vi "8HP_EnFlo_Specific.vi"(2 "Datalog file path (full)":path, 3 "COM port":refnum<visa-resource-name>, 4 "Log data stream":bool, 5 "Set data rate (Hz)":u8(ring)=14 items=["1", "2", "4", "5", "8", "10", "16", "20", "25", "32", "40", "50", "64", "80", "100", "125", "160", "200", "250", "320", "400", "500", "625", "800", "1000"], 6 "N samples":u32=1000, 7 "Command":T2="s") -> (0 "Error":errorcluster, 1 "All samples out":sgl[][](array[numeric]))   [LabVIEW 2020]
uses:
  ctls/8HP_Cmd (USB).ctl
  Globals/Meas_global.vi
panel:
  in  "Main":T1(tab)
  out "Serial number":sgl
  out "Subsystems ok":bool[](array[boolean])
  out "Pressure sensor values in range":bool[](array[boolean])
  out "Pressure sensor temperatures in range":bool[](array[boolean])
  out "Pressure sensor EEPROM checksums ok":bool[](array[boolean])
  out "P_raw_Azero":sgl[](array[numeric])
  out "n":u16
  out "Auto zero progBar":u16(slide) caption="Collecting samples, please maintain dP = 0" scale=0.0..1000.0
  in  "EEPROM array 2":u16[](array[numeric])
  in  "EEPROM array":sgl[](array[numeric])
  out "Chk ok":bool
  out "EEPROM Checksum":u8 format="%02x"
  out "received":bool
  out "Returned data rate (Hz)":u16
  out "sent":bool
  in  "Stop Data":bool
  out "Relative humidity (%)":sgl
  out "Env. sensor die temperature (deg C)":sgl
  out "External thermistor 0 temperature (deg C)":sgl
  out "Atmospheric pressure (mbar)":sgl
  out "Checksum ok":bool
  out "Gyration vector (deg / s)":sgl[](array[numeric])
  out "Acceleration vector (g)":sgl[](array[numeric])
  out "Pressures":sgl[][](graph)
  out "Stream enabled":bool
  out "External thermistor 1 temperature (deg C)":sgl
  # "Paul Nathan 10/2018"
  # "Output array order:\nP0 (Pa)\n  |\nP7 (Pa)\nT0 (deg C)\nT1 (deg C)\nP_atmos (mbar)\nT_env (deg C)\nRH (%)\nax (g)\nay (g)\naz (g)\nwx (deg / s)\nwy (deg / s)\nwz (deg / s)"
  # "Environmental sensor present"
  # "Inertial sensor present"
  # "Accelerometer self test pass"
  # "Gyroscope self test pass"
  # "External thermistor 0 value in range"
  # "External thermistor 1 value in range"
  # "MCU EEPROM checksum ok"
  # "Pressure sensor 0 value in range"
  # "Pressure sensor 1 value in range"
  # "Pressure sensor 2 value in range"
  # "Pressure sensor 3 value in range"
  # "Pressure sensor 4 value in range"
  # "Pressure sensor 5 value in range"
  # "Pressure sensor 6 value in range"
  # "Pressure sensor 7 value in range"
  # "Pressure sensor 0 temperature in range"
  # "Pressure sensor 1 temperature in range"
  # "Pressure sensor 2 temperature in range"
  # "Pressure sensor 3 temperature in range"
  # "Pressure sensor 4 temperature in range"
  # "Pressure sensor 5 temperature in range"
  # "Pressure sensor 6 temperature in range"
  # "Pressure sensor 7 temperature in range"
  # "Pressure sensor 0 EEPROM checksum okay"
  # "Pressure sensor 1 EEPROM checksum okay"
  # "Pressure sensor 2 EEPROM checksum okay"
  # "Pressure sensor 3 EEPROM checksum okay"
  # "Pressure sensor 4 EEPROM checksum okay"
  # "Pressure sensor 5 EEPROM checksum okay"
  # "Pressure sensor 6 EEPROM checksum okay"
  # "Pressure sensor 7 EEPROM checksum okay"
  # "of 1000"
  # "P0 raw auto-zero"
  # "P1 raw auto-zero"
  # "P2 raw auto-zero"
  # "P3 raw auto-zero"
  # "P4 raw auto-zero"
  # "P5 raw auto-zero"
  # "P6 raw auto-zero"
  # "P7 raw auto-zero"
  # "Power-up defaults"
  # "Data rate (Hz)"
  # "TTL streaming"
  # "USB streaming"
  # "TTL stream contains full data"
  # "Accelerometer range mode"
  # "Gyroscope range mode"
  # "IMU rate mode"
  # "P0 raw auto-zero"
  # "P1 raw auto-zero"
  # "P2 raw auto-zero"
  # "P3 raw auto-zero"
  # "P4 raw auto-zero"
  # "P5 raw auto-zero"
  # "P6 raw auto-zero"
  # "P7 raw auto-zero"
  # "Atmospheric pressure offset (Pa)"
  # "External thermistor 0 temperature offset (deg C)"
  # "External thermistor 1 temperature offset (deg C)"
  # "Serial number"
  # "Baud rate (bps)"
  # "Accelerometer vector magnitude scale factor"
  # "Gyroscope x component offset (deg / s)"
  # "Gyroscope y component offset (deg / s)"
  # "Gyroscope z component offset (deg / s)"
  # "w_x"
  # "w_y"
  # "w_z"
  # "a_x"
  # "a_y"
  # "a_z"
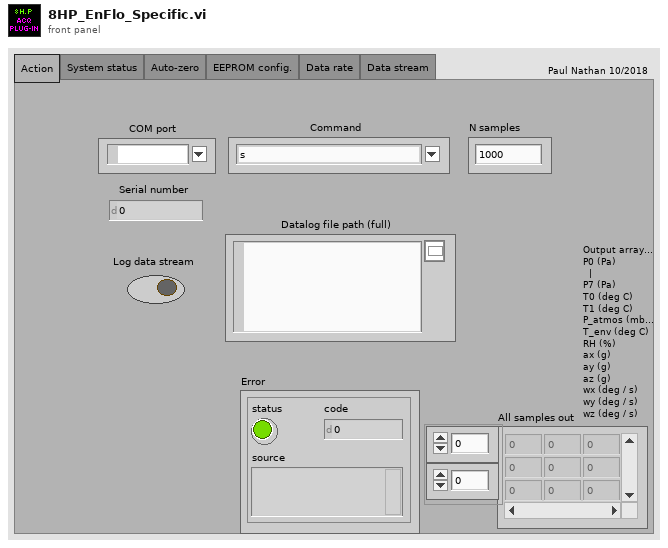
[diagram p1: front panel]
types:
  T1 = enum32{"Action", "System status", "Auto-zero", "EEPROM config.", "Data rate", "Data stream"}
  T2 = typedef "8HP_Cmd (USB).ctl" = string
  T3 = enum16{"open", "replace", "create", "open or create", "replace or create", "replace or create with confirmation"}
  T4 = typedef "Rendezvous RefNum" = refnum<k1>
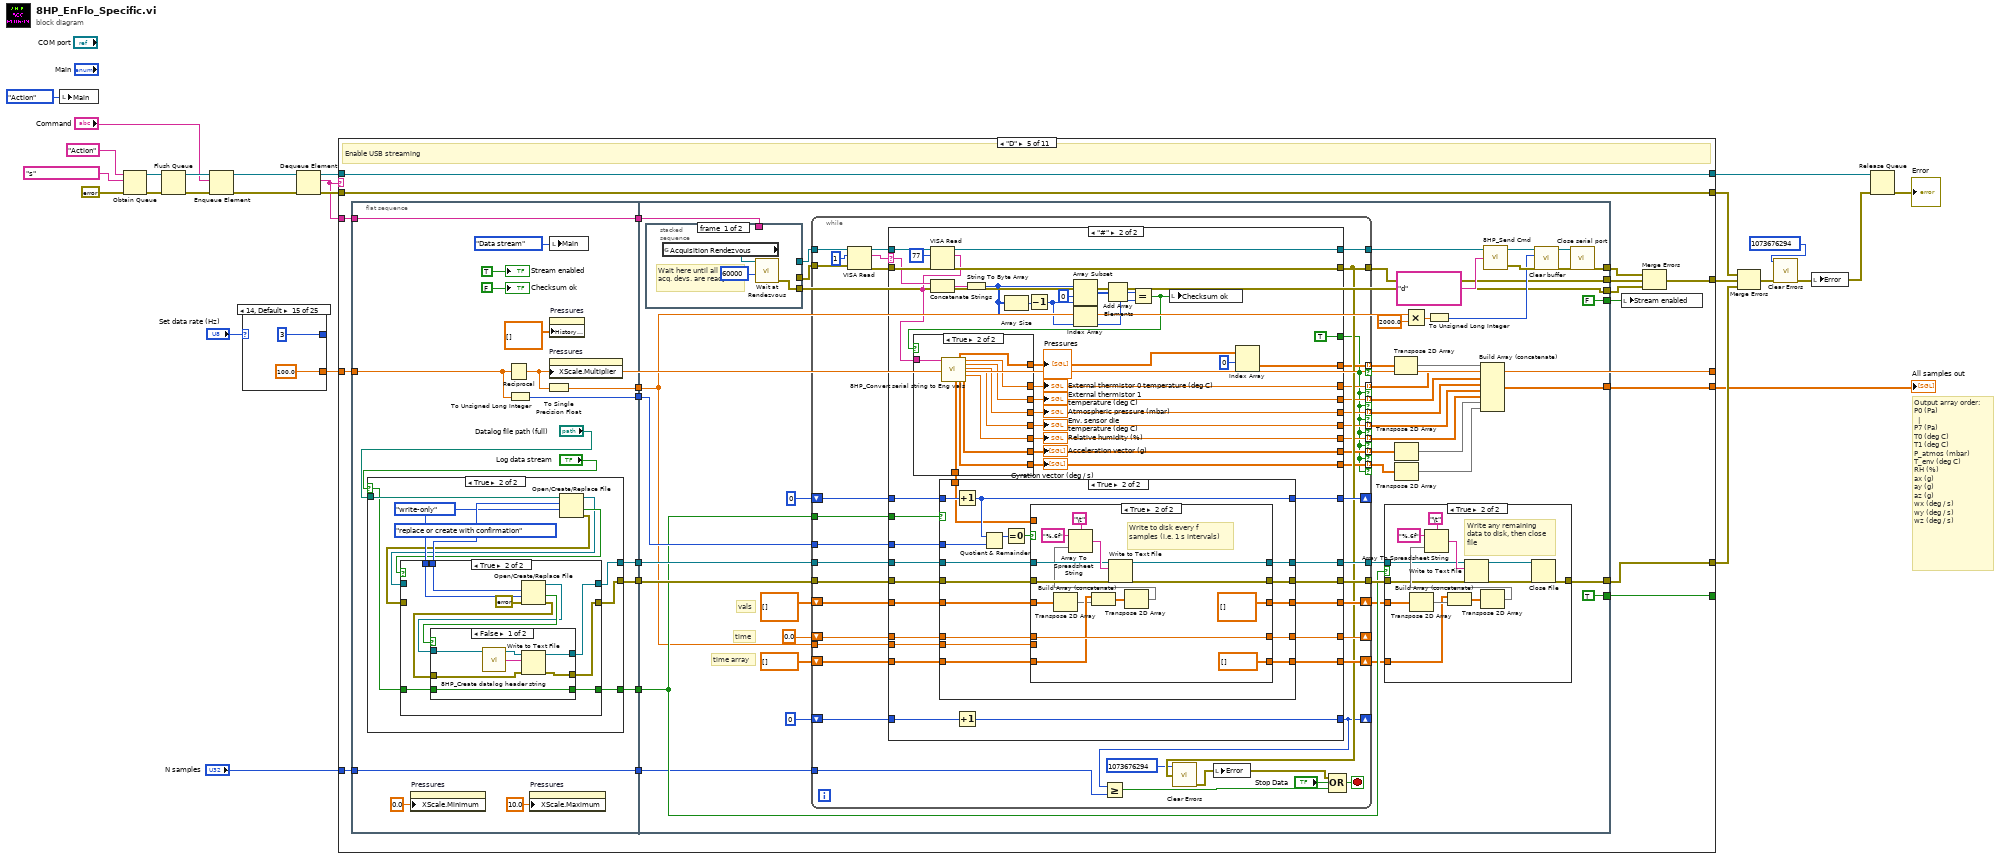
[diagram p0: block diagram]
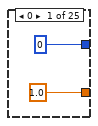
[diagram p2: hidden frame]
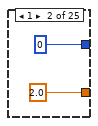
[diagram p3: hidden frame]
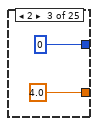
[diagram p4: hidden frame]
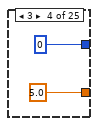
[diagram p5: hidden frame]
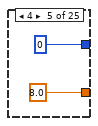
[diagram p6: hidden frame]
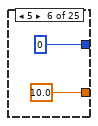
[diagram p7: hidden frame]
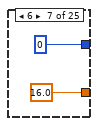
[diagram p8: hidden frame]
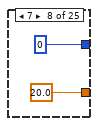
[diagram p9: hidden frame]
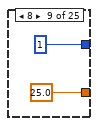
[diagram p10: hidden frame]
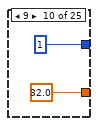
[diagram p11: hidden frame]
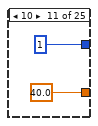
[diagram p12: hidden frame]
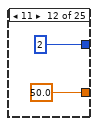
[diagram p13: hidden frame]
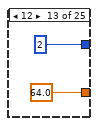
[diagram p14: hidden frame]
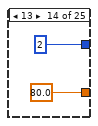
[diagram p15: hidden frame]
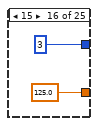
[diagram p16: hidden frame]
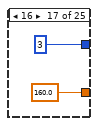
[diagram p17: hidden frame]
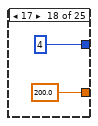
[diagram p18: hidden frame]
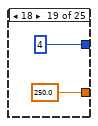
[diagram p19: hidden frame]
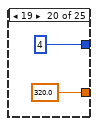
[diagram p20: hidden frame]
diagram:
  # "Output array order:\nP0 (Pa)\n  |\nP7 (Pa)\nT0 (deg C)\nT1 (deg C)\nP_atmos (mbar)\nT_env (deg C)\nRH (%)\nax (g)\nay (g)\naz (g)\nwx (deg / s)\nwy (deg / s)\nwz (deg / s)"
  n1 = local write "Main"(T1."Action" ("Main")) -> ()
  n2 = Obtain Queue(name (unnamed)="Action", element data type=T2 "s" ("Combo Box"), error in (no error)=errorcluster {"status"=FALSE, "code"=0, "source"=""}) -> (queue out=w24:refnum<queue>, error out=w25:errorcluster)  [unwired: 2 in, 1 out]
  n3 = Flush Queue(queue=w24, error in (no error)=w25) -> (queue out=w17:refnum<queue>, error out=w16:errorcluster)  [unwired: 1 out]
  n4 = Enqueue Element(queue=w17, element="Command", error in (no error)=w16) -> (queue out=w19:refnum<queue>, error out=w18:errorcluster)  [unwired: 1 in, 1 out]
  n5 = case shown="14, Default" "Set data rate (Hz)" {
    tunnel: [1.0 2.0 4.0 5.0 8.0 10.0 16.0 20.0 25.0 32.0 40.0 50.0 64.0 80.0 100.0 125.0 160.0 200.0 250.0 320.0 400.0 500.0 625.0 800.0 1000.0] -> w4
    tunnel: [u8 0 u8 0 u8 0 u8 0 u8 0 u8 0 u8 0 u8 0 u8 1 u8 1 u8 1 u8 2 u8 2 u8 2 u8 3 u8 3 u8 3 u8 4 u8 4 u8 4 u8 5 u8 5 u8 6 u8 6 u8 6] -> _
    frame 0 {
    }
    frame 1 {
    }
    frame 2 {
    }
    frame 3 {
    }
    frame 4 {
    }
    frame 5 {
    }
    frame 6 {
    }
    frame 7 {
    }
    frame 8 {
    }
    frame 9 {
    }
    frame 10 {
    }
    frame 11 {
    }
    frame 12 {
    }
    frame 13 {
    }
    frame 14, Default {
    }
    frame 15 {
    }
    frame 16 {
    }
    frame 17 {
    }
    frame 18 {
    }
    frame 19 {
    }
    frame 20 {
    }
    frame 21 {
    }
    frame 22 {
    }
    frame 23 {
    }
    frame 24 {
    }
  }
  n6 = Dequeue Element(queue=w19, error in (no error)=w18) -> (queue out=w14:refnum<queue>, element=w12:T2, error out=w13:errorcluster)  [unwired: 1 in, 1 out]
  n7 = case shown="\"D\"" w12 {
    tunnel: [w83 w124 w163 w239 w317 w607 w633 w716 w756 FALSE FALSE] -> _
    tunnel: w14 -> [w82 w123 w162 w238 w316 w609 w635 w718 w755 w780 w785]
    tunnel: [w82 w123 w162 w238 w316 w609 w635 w718 w755 w780 w785] -> w6
    tunnel: w13 -> [w81 w122 w161 w237 w315 w608 w636 w719 w754 w779 w784]
    tunnel: [w81 w122 w161 w237 w315 w608 w636 w719 w754 w779 w784] -> w11
    tunnel: w12 -> [w80 w121 w160 w236 w314 w611 w641 w724 w753 _ _]
    tunnel: [w78 w119 w158 w233 w300 w610 w634 w717 w751 errorcluster {"status"=FALSE, "code"=0, "source"=""} ("Error out") errorcluster {"status"=FALSE, "code"=0, "source"=""} ("Error out")] -> w10
    tunnel: [_ _ _ _ w312 _ _ _ _ _ _] -> w9
    tunnel: w4 -> [w77 w118 w157 w232 w305 w605 _ _ w750 w776 w781]
    tunnel: [w77 w118 w157 w232 w305 w605 w637 w720 w750 w776 w781] -> _
    tunnel: [_ _ _ _ w304 _ _ _ _ _ _] -> w2
    tunnel: "N samples" -> [_ _ _ _ w298 _ _ _ _ _ _]
    frame "S", "s" {
      # "Perform self-test and retrieve status bytes, Retrieve status bytes"
      n8 = flat-sequence {
        tunnel: w80 -> [w86]
        tunnel: [w86] -> w79
        tunnel: [TRUE] -> w83
        tunnel: w79 -> [w92]
        tunnel: [w87] -> w78
        frame #0 {
          w85 = bool[] [] ("Pressure sensor EEPROM checksums ok")
          n9 = local write "Main"(T1."System status" ("Main")) -> ()
          "Pressure sensor EEPROM checksums ok" <- w85
          "Pressure sensor temperatures in range" <- w85
          "Pressure sensor values in range" <- w85
          "Subsystems ok" <- w85
        }
        frame #1 {
          w97 = 1 ("length (rest)")
          w105 = u8 0 ("byte count")
          n10 = local read "COM port"() -> (w93:refnum<visa-resource-name>)
          n11 = call "Open serial port.vi"("timeout (ms)"=u32 5000, "VISA resource name"=w93) -> ("Error out"=w115:errorcluster, "VISA resource name out"=w116:refnum<visa-resource-name>)  [unwired: 8 in]
          n12 = call "8HP_Send Cmd.vi"("Error In"=w115, "Operation"=w92, "Port"=w116) -> ("Error Out"=w113:errorcluster, "Port out"=w114:refnum<visa-resource-name>)  [unwired: 1 in]
          n13 = VISA Read(VISA resource name=w114, byte count=u32 4, error in (no error)=w113) -> (VISA resource name out=w111:refnum<visa-resource-name>, read buffer=w100:string, error out=w110:errorcluster)  [unwired: 1 out]
          n14 = call "Close serial port.vi"("Error in"=w110, "VISA resource name"=w111) -> ("Error out"=w87:errorcluster)  [unwired: 9 in]
          n15 = String Subset(string=w100, offset (0)=0, length (rest)=w97) -> (substring=w109:string)
          n16 = String Subset(string=w100, offset (0)=1, length (rest)=w97) -> (substring=w108:string)
          n17 = String Subset(string=w100, offset (0)=2 ("length (rest)"), length (rest)=w97) -> (substring=w107:string)
          n18 = String Subset(string=w100, offset (0)=3, length (rest)=w97) -> (substring=w106:string)
          n19 = Type Cast(type=w105, x=w109) -> (*(type *) &x=w104:u8)
          n20 = Type Cast(type=w105, x=w108) -> (*(type *) &x=w103:u8)
          n21 = Type Cast(type=w105, x=w107) -> (*(type *) &x=w102:u8)
          n22 = Type Cast(type=w105, x=w106) -> (*(type *) &x=w101:u8)
          n23 = Number To Boolean Array(number=w104) -> (Boolean array=w91:bool[])
          n24 = Number To Boolean Array(number=w103) -> (Boolean array=w90:bool[])
          n25 = Number To Boolean Array(number=w102) -> (Boolean array=w89:bool[])
          n26 = Number To Boolean Array(number=w101) -> (Boolean array=w88:bool[])
          n27 = local write "Pressure sensor EEPROM checksums ok"(w91) -> ()
          n28 = local write "Pressure sensor temperatures in range"(w90) -> ()
          n29 = local write "Pressure sensor values in range"(w89) -> ()
          n30 = local write "Subsystems ok"(w88) -> ()
        }
      }
    }
    frame "Z", "z" {
      # "Perform permanent auto-zero (write values to EEPROM), Perform temporary auto-zero"
      n31 = flat-sequence {
        tunnel: w121 -> [w128]
        tunnel: [w128] -> w120
        tunnel: [TRUE] -> w124
        tunnel: w120 -> [w135]
        tunnel: [w131] -> w119
        frame #0 {
          n32 = local write "Main"(T1."Auto-zero" ("Main")) -> ()
          "P_raw_Azero" <- sgl[] [] ("P_raw_Azero")
          "Auto zero progBar" <- u16 0 ("Collecting samples, please maintain dP = 0")
        }
        frame #1 {
          n33 = local read "COM port"() -> (w136:refnum<visa-resource-name>)
          n34 = call "Open serial port.vi"("timeout (ms)"=u32 16000, "VISA resource name"=w136) -> ("Error out"=w143:errorcluster, "VISA resource name out"=w144:refnum<visa-resource-name>)  [unwired: 8 in]
          n35 = call "8HP_Send Cmd.vi"("Error In"=w143, "Operation"=w135, "Port"=w144) -> ("Error Out"=w141:errorcluster, "Port out"=w142:refnum<visa-resource-name>)  [unwired: 1 in]
          n36 = VISA Read(VISA resource name=w142, byte count=u32 32, error in (no error)=w141) -> (VISA resource name out=w139:refnum<visa-resource-name>, read buffer=w132:string, error out=w138:errorcluster)  [unwired: 1 out]
          n37 = for {
            N: 1000 -> [_]
            shift-right: [w146] -> _
            shift-left: u16 0 -> [w147]
            n38 = Increment(x=w147) -> (x+1=w146:u16)
            "n" <- w146
            n39 = Wait (ms)(milliseconds to wait=u32 10) -> ()  [unwired: 1 out]
            n40 = local write "Auto zero progBar"(w146) -> ()
          }
          n41 = for {
            N: 8 -> [_]
            tunnel: [w150] -> w134 mode=indexing
            tunnel: w132 -> [w149]
            i -> [w156]
            w154 = 4 ("x")
            # "to BE"
            n42 = Multiply(x=w154, y=w156) -> (x*y=w155:i32)
            n43 = String Subset(string=w149, offset (0)=w155, length (rest)=w154) -> (substring=w153:string)
            n44 = Reverse String(1:w153) -> (0:w152:string)
            n45 = Type Cast(type=sgl 0.0 ("byte count"), x=w152) -> (*(type *) &x=w150:sgl)
          }
          n46 = call "Close serial port.vi"("Error in"=w138, "VISA resource name"=w139) -> ("Error out"=w131:errorcluster)  [unwired: 9 in]
          n47 = local write "P_raw_Azero"(w134) -> ()
        }
      }
    }
    frame "R" {
      # "Read all EEPROM values"
      n48 = flat-sequence {
        tunnel: w160 -> [w167]
        tunnel: [w167] -> w159
        tunnel: [TRUE] -> w163
        tunnel: w159 -> [w202]
        tunnel: [w191] -> w158
        frame #0 {
          n49 = local write "EEPROM array"(sgl[] [] ("EEPROM array")) -> ()
          n50 = local write "EEPROM array 2"(u16[] [] ("EEPROM array 2")) -> ()
          n51 = local write "Main"(T1."EEPROM config." ("Main")) -> ()
        }
        frame #1 {
          # "to BE"
          n52 = local read "COM port"() -> (w203:refnum<visa-resource-name>)
          n53 = call "Open serial port.vi"("timeout (ms)"=u32 5000, "VISA resource name"=w203) -> ("Error out"=w210:errorcluster, "VISA resource name out"=w211:refnum<visa-resource-name>)  [unwired: 8 in]
          n54 = call "8HP_Send Cmd.vi"("Error In"=w210, "Operation"=w202, "Port"=w211) -> ("Error Out"=w208:errorcluster, "Port out"=w209:refnum<visa-resource-name>)  [unwired: 1 in]
          n55 = VISA Read(VISA resource name=w209, byte count=u32 78, error in (no error)=w208) -> (VISA resource name out=w206:refnum<visa-resource-name>, read buffer=w174:string, error out=w205:errorcluster)  [unwired: 1 out]
          n56 = String To Byte Array(string=w174) -> (unsigned byte array=w194:u8[])
          n57 = call "Close serial port.vi"("Error in"=w205, "VISA resource name"=w206) -> ("Error out"=w191:errorcluster)  [unwired: 9 in]
          n58 = String Subset(string=w174, offset (0)=0, length (rest)=56 ("length (rest)")) -> (substring=w189:string)
          n59 = String Subset(string=w174, offset (0)=64, length (rest)=12 ("length (rest)")) -> (substring=w184:string)
          n60 = String Subset(string=w174, offset (0)=56, length (rest)=2 ("length (rest)")) -> (substring=w173:string)
          n61 = String Subset(string=w174, offset (0)=58, length (rest)=6 ("length (rest)")) -> (substring=w168:string)
          n62 = Array Size(array=w194) -> (size(s)=w196:i32)
          n63 = Decrement(x=w196) -> (x-1=w195:i32)
          n64 = for {
            N: 14 -> [_]
            tunnel: [w224] -> w183 mode=indexing
            tunnel: w189 -> [w223]
            i -> [w228]
            w226 = 4 ("x")
            # "to BE"
            n65 = Multiply(x=w226, y=w228) -> (x*y=w227:i32)
            n66 = String Subset(string=w223, offset (0)=w227, length (rest)=w226) -> (substring=w222:string)
            n67 = Reverse String(1:w222) -> (0:w221:string)
            n68 = Type Cast(type=sgl 0.0 ("byte count"), x=w221) -> (*(type *) &x=w224:sgl)
          }
          n69 = for {
            N: 3 -> [_]
            tunnel: [w216] -> w182 mode=indexing
            tunnel: w184 -> [w215]
            i -> [w220]
            w218 = 4 ("x")
            # "to BE"
            n70 = Multiply(x=w218, y=w220) -> (x*y=w219:i32)
            n71 = String Subset(string=w215, offset (0)=w219, length (rest)=w218) -> (substring=w214:string)
            n72 = Reverse String(1:w214) -> (0:w213:string)
            n73 = Type Cast(type=sgl 0.0 ("byte count"), x=w213) -> (*(type *) &x=w216:sgl)
          }
          n74 = Index Array(array=w194, index=77) -> (element=w198:u8)
          n75 = Array Subset(array=w194, index=0, length=w195) -> (w192:u8[])
          n76 = Reverse String(1:w173) -> (0:w180:string)
          n77 = Add Array Elements(numeric array=w192) -> (sum=w193:u8)
          n78 = Type Cast(type=u16 0 ("byte count"), x=w180) -> (*(type *) &x=w172:u16)
          n79 = String To Byte Array(string=w168) -> (unsigned byte array=w171:u8[])
          n80 = To Unsigned Word Integer(number=w171) -> (unsigned 16bit integer=w169:u16[])
          n81 = Equal?(x=w198, y=w193) -> (x = y?=w200:bool)
          n82 = Build Array (concatenate)(w183, w182) -> (w181:sgl[])
          n83 = Build Array (concatenate)(w172, w169) -> (w170:u16[])
          n84 = local write "EEPROM array"(w181) -> ()
          n85 = local write "EEPROM array 2"(w170) -> ()
          n86 = local write "EEPROM Checksum"(w198) -> ()
          n87 = local write "Chk ok"(w200) -> ()
        }
      }
    }
    frame "W" {
      # "Write all EEPROM values (including new checksum)"
      n88 = flat-sequence {
        tunnel: w236 -> [w252]
        tunnel: [w252] -> w235
        tunnel: [w246] -> w234
        tunnel: [w245] -> w231
        tunnel: [w241] -> w230
        tunnel: [w242] -> w229
        tunnel: [TRUE] -> w239
        tunnel: w235 -> [w280]
        tunnel: w234 -> [w274]
        tunnel: [w272] -> w233
        tunnel: w231 -> [w261]
        tunnel: w230 -> [w258]
        tunnel: w229 -> [w256]
        frame #0 {
          n89 = local write "Main"(T1."EEPROM config." ("Main")) -> ()
          n90 = Split 1D Array(array="EEPROM array", index=14) -> (first subarray=w246:sgl[], second subarray=w245:sgl[])
          n91 = Split 1D Array(array="EEPROM array 2", index=1) -> (first subarray=w244:u16[], second subarray=w243:u16[])
          n92 = Index Array(array=w244, index=0) -> (element=w241:u16)
          n93 = To Unsigned Byte Integer(number=w243) -> (unsigned 8bit integer=w242:u8[])
        }
        frame #1 {
          # "to LE"
          n94 = local read "COM port"() -> (w281:refnum<visa-resource-name>)
          n95 = for {
            N: 14 -> [_]
            tunnel: w274 -> [w294] mode=indexing
            shift-right: [w295] -> w267
            shift-left: "" -> [w296]
            # "to LE"
            n96 = Type Cast(type="", x=w294) -> (*(type *) &x=w293:string)
            n97 = Reverse String(1:w293) -> (0:w292:string)
            n98 = Concatenate Strings(w296, w292) -> (w295:string)
          }
          n99 = for {
            N: 3 -> [_]
            tunnel: w261 -> [w288] mode=indexing
            shift-right: [w289] -> w254
            shift-left: "" -> [w290]
            # "to LE"
            n100 = Type Cast(type="", x=w288) -> (*(type *) &x=w287:string)
            n101 = Reverse String(1:w287) -> (0:w286:string)
            n102 = Concatenate Strings(w290, w286) -> (w289:string)
          }
          n103 = Type Cast(type="", x=w258) -> (*(type *) &x=w260:string)
          n104 = Reverse String(1:w260) -> (0:w257:string)
          n105 = Byte Array To String(unsigned byte array=w256) -> (string=w253:string)
          n106 = call "Open serial port.vi"("timeout (ms)"=u32 5000, "VISA resource name"=w281) -> ("Error out"=w283:errorcluster, "VISA resource name out"=w284:refnum<visa-resource-name>)  [unwired: 8 in]
          n107 = Type Cast(type="", x=u8 0) -> (*(type *) &x=w255:string)
          n108 = Concatenate Strings(w267, w257, w253, w254, w255) -> (w264:string)
          n109 = String To Byte Array(string=w264) -> (unsigned byte array=w268:u8[])
          n110 = Add Array Elements(numeric array=w268) -> (sum=w273:u8)
          "EEPROM Checksum" <- w273
          n111 = Type Cast(type="", x=w273) -> (*(type *) &x=w276:string)
          n112 = Concatenate Strings(w264, w276) -> (w271:string)
          n113 = call "8HP_Send Cmd + Data.vi"("Error In"=w283, "Data"=w271, "Operation"=w280, "Port"=w284) -> ("Error Out"=w269:errorcluster, "Port out"=w270:refnum<visa-resource-name>)  [unwired: 1 in]
          n114 = call "Close serial port.vi"("Error in"=w269, "VISA resource name"=w270) -> ("Error out"=w272:errorcluster)  [unwired: 9 in]
          "Chk ok" <- TRUE ("Chk ok")
        }
      }
    }
    frame "D" {
      # "Enable USB streaming"
      n115 = flat-sequence {
        tunnel: w314 -> [w334]
        tunnel: [w334] -> w313
        tunnel: [w331] -> w311
        tunnel: [w330] -> w310
        tunnel: [w329] -> w309
        tunnel: w305 -> [w320]
        tunnel: [w327] -> w308
        tunnel: [w323] -> w307
        tunnel: [w321] -> w299
        tunnel: w298 -> [w321]
        tunnel: [TRUE] -> w317
        tunnel: w313 -> [w389]
        tunnel: [w416] -> w302
        tunnel: [w415] -> w312
        tunnel: w311 -> [w412]
        tunnel: w310 -> [w411]
        tunnel: w309 -> [w413]
        tunnel: w308 -> [w395]
        tunnel: w307 -> [w405]
        tunnel: [FALSE] -> w306
        tunnel: [w385] -> w304
        tunnel: [w373] -> w301
        tunnel: [w376] -> w303
        tunnel: w299 -> [w375]
        frame #0 {
          n116 = case shown="True" "Log data stream" {
            selector: "Log data stream" -> [w335 w338]
            tunnel: "Datalog file path (full)" -> [_ w347]
            tunnel: [refnum<file> refnum ("refnum out") w344] -> w331
            tunnel: [errorcluster {"status"=FALSE, "code"=0, "source"=""} ("error out") w343] -> w330
            tunnel: [w335 w339] -> w323
            frame False {
            }
            frame True {
              w345 = enum16{"read/write", "read-only", "write-only"}."write-only" ("access (0:read/write)")
              w346 = T3."replace or create with confirmation" ("operation (0:open)")
              n117 = Open/Create/Replace File(file path (use dialog)=w347, operation (0:open)=w346, access (0:read/write)=w345) -> (refnum out=w340:refnum<file>, cancelled=w342:bool, error out=w341:errorcluster)  [unwired: 3 in]
              n118 = case shown="True" w342 {
                tunnel: w346 -> [_ w363]
                tunnel: w345 -> [_ w362]
                tunnel: w341 -> [w351 _]
                tunnel: [w349 w357] -> w344
                tunnel: [w350 w358] -> w343
                tunnel: w340 -> [w352 _]
                tunnel: [w348 w355] -> w339
                tunnel: w338 -> [w348 w354]
                frame False {
                  n119 = call "8HP_Create datalog header string.vi"() -> ("Datalog header string"=w353:string)  [unwired: 1 in]
                  n120 = Write to Text File(file (use dialog)=w352, text=w353, error in=w351) -> (refnum out=w349:refnum<file>, error out=w350:errorcluster)  [unwired: 1 in, 1 out]
                }
                frame True {
                  n121 = Open/Create/Replace File(error in=errorcluster {"status"=FALSE, "code"=0, "source"=""}, operation (0:open)=w363, access (0:read/write)=w362) -> (refnum out=w360:refnum<file>, cancelled=w361:bool, error out=w359:errorcluster)  [unwired: 3 in]
                  n122 = case shown="False" w361 {
                    tunnel: w360 -> [w368 _]
                    tunnel: w359 -> [w367 _]
                    tunnel: [w366 errorcluster {"status"=FALSE, "code"=0, "source"=""} ("error out")] -> w358
                    tunnel: [w365 refnum<file> refnum ("t")] -> w357
                    tunnel: [w364 w370] -> w355
                    tunnel: w354 -> [w364 _]
                    frame False {
                      n123 = call "8HP_Create datalog header string.vi"() -> ("Datalog header string"=w369:string)  [unwired: 1 in]
                      n124 = Write to Text File(file (use dialog)=w368, text=w369, error in=w367) -> (refnum out=w365:refnum<file>, error out=w366:errorcluster)  [unwired: 1 in, 1 out]
                    }
                    frame True {
                      w370 = FALSE ("Log data stream")
                      n125 = local write "Log data stream"(w370) -> ()
                    }
                  }
                }
              }
            }
          }
          n126 = property on="Pressures" class="WFChart (strict)"("XScale.Minimum"=0.0 ("X Scale.Range:Minimum")) -> ()  [unwired: 2 in, 2 out]
          n127 = Reciprocal(x=w320) -> (1/x=w328:dbl)
          n128 = To Unsigned Long Integer(number=w320) -> (unsigned 32bit integer=w329:u32)
          n129 = property on="Pressures" class="WFChart (strict)"("XScale.Maximum"=10.0 ("X Scale.Range:Minimum")) -> ()  [unwired: 2 in, 2 out]
          n130 = To Single Precision Float(number=w328) -> (single precision float=w327:sgl)
          n131 = property on="Pressures" class="WFChart (strict)"("XScale.Multiplier"=w328) -> ()  [unwired: 2 in, 2 out]
          n132 = local write "Main"(T1."Data stream" ("Main")) -> ()
          n133 = property on="Pressures" class="WFChart (strict)"("History Data"=sgl[][] []) -> ()  [unwired: 2 in, 2 out]
          "Checksum ok" <- FALSE ("Checksum ok")
          "Stream enabled" <- TRUE ("Stream enabled")
        }
        frame #1 {
          # "vals"
          # "time"
          # "time array"
          n134 = stacked-sequence {
            tunnel: [_ w425] -> w404
            tunnel: [_ w423] -> w403
            tunnel: w389 -> [_ w421]
            tunnel: [w419 _] -> w373
            frame #0 {
              # "Wait here until all acq. devs. are ready."
              n135 = global read "Meas_global.vi" "Acquisition Rendezvous"() -> (w420:T4)
              n136 = call <vilib>:"Wait at Rendezvous.vi"("ms timeout (-1)"=60000, "rendezvous"=w420) -> ("error out"=w419:errorcluster)  [unwired: 3 in, 2 out]
            }
            frame #1 {
              n137 = local read "COM port"() -> (w427:refnum<visa-resource-name>)
              n138 = call "Open serial port.vi"("timeout (ms)"=u32 5000, "VISA resource name"=w427) -> ("Error out"=w424:errorcluster, "VISA resource name out"=w426:refnum<visa-resource-name>)  [unwired: 8 in]
              n139 = call "8HP_Send Cmd.vi"("Error In"=w424, "Operation"=w421, "Port"=w426) -> ("Error Out"=w423:errorcluster, "Port out"=w425:refnum<visa-resource-name>)  [unwired: 1 in]
            }
          }
          n140 = while {
            tunnel: [w457] -> w376
            tunnel: w404 -> [w459]
            tunnel: [w477] -> w402
            shift-right: [w473] -> _
            shift-left: u32 0 -> [w474]
            tunnel: w413 -> [w472]
            tunnel: w412 -> [w471]
            tunnel: w411 -> [w470]
            tunnel: [w469] -> w410
            tunnel: [w468] -> w409
            shift-right: [w467] -> w392
            shift-left: sgl[][] [] -> [w466]
            shift-right: [w463] -> _
            shift-left: sgl 0.0 ("Numeric") -> [w465]
            tunnel: w395 -> [w464]
            shift-right: [w461] -> w391
            shift-left: sgl[] [] -> [w462]
            tunnel: w405 -> [w460]
            tunnel: w403 -> [w458]
            tunnel: [w454] -> w384 mode=indexing if=w446
            tunnel: [w453] -> w383 mode=indexing if=w446
            tunnel: [w452] -> w382 mode=indexing if=w446
            tunnel: [w451] -> w381 mode=indexing if=w446
            tunnel: [w450] -> w380 mode=indexing if=w446
            tunnel: [w449] -> w377 mode=indexing if=w446
            tunnel: [w448] -> w378 mode=indexing if=w446
            tunnel: [w447] -> w379 mode=indexing if=w446
            tunnel: w375 -> [w444]
            shift-right: [w442] -> _
            shift-left: u32 0 -> [w445]
            stop <- w475 stop-if-true
            n141 = VISA Read(VISA resource name=w459, byte count=u32 1, error in (no error)=w458) -> (VISA resource name out=w479:refnum<visa-resource-name>, read buffer=w480:string, error out=w478:errorcluster)  [unwired: 1 out]
            n142 = case shown="\"#\"" w480 {
              selector: w480 -> [_ w531]
              tunnel: w479 -> [w490 w535]
              tunnel: [w491 w533] -> w457
              tunnel: w478 -> [w491 w536]
              tunnel: [w490 w534] -> w477
              tunnel: w474 -> [w489 w521]
              tunnel: [w489 w520] -> w473
              tunnel: w472 -> [_ w519]
              tunnel: w471 -> [w488 w518]
              tunnel: w470 -> [w487 w517]
              tunnel: [w487 w516] -> w469
              tunnel: [w488 w515] -> w468
              tunnel: [w486 w514] -> w467
              tunnel: w466 -> [w486 w513]
              tunnel: w465 -> [w485 w512]
              tunnel: w464 -> [_ w511]
              tunnel: [w485 w510] -> w463
              tunnel: w462 -> [w484 w509]
              tunnel: [w484 w508] -> w461
              tunnel: w460 -> [_ w507]
              tunnel: [_ w506] -> w454
              tunnel: [FALSE TRUE] -> w446
              tunnel: [_ w492] -> w453
              tunnel: [_ w493] -> w452
              tunnel: [_ w494] -> w451
              tunnel: [_ w500] -> w450
              tunnel: [_ w499] -> w449
              tunnel: [_ w498] -> w448
              tunnel: [_ w497] -> w447
              tunnel: w445 -> [w482 w496]
              tunnel: [w482 w495] -> w442
              frame Default {
              }
              frame "#" {
                n143 = VISA Read(VISA resource name=w535, byte count=u32 77, error in (no error)=w536) -> (VISA resource name out=w534:refnum<visa-resource-name>, read buffer=w522:string, error out=w533:errorcluster)  [unwired: 1 out]
                n144 = Concatenate Strings(w531, w522) -> (w523:string)
                n145 = Increment(x=w496) -> (x+1=w495:u32)
                n146 = String To Byte Array(string=w523) -> (unsigned byte array=w526:u8[])
                n147 = Array Size(array=w526) -> (size(s)=w529:i32)
                n148 = Decrement(x=w529) -> (x-1=w525:i32)
                n149 = Array Subset(array=w526, index=0, length=w525) -> (w530:u8[])
                n150 = Index Array(array=w526, index=w525) -> (element=w524:u8)
                n151 = Add Array Elements(numeric array=w530) -> (sum=w527:u8)
                n152 = Equal?(x=w527, y=w524) -> (x = y?=w502:bool)
                n153 = case shown="True" w502 {
                  tunnel: w522 -> [_ w556]
                  tunnel: [w546 w555] -> w492
                  tunnel: [w546 w554] -> w493
                  tunnel: [w546 w553] -> w500
                  tunnel: [w546 w552] -> w499
                  tunnel: [w544 w551] -> w498
                  tunnel: [w544 w550] -> w497
                  tunnel: [w541 w549] -> w505
                  tunnel: [w546 w548] -> w494
                  tunnel: [w537 w547] -> w503
                  frame False {
                    (unwired) 3 ("dimension size")
                    w546 = sgl nan ("Atmospheric pressure (mbar)")
                    n154 = Initialize Array(sgl nan ("element"), 8 ("dimension size")) -> (w540:sgl[])
                    n155 = Initialize Array(sgl nan ("element")) -> (w544:sgl[])  [unwired: 1 in]
                    n156 = Initialize Array(sgl nan ("element"), 19 ("dimension size")) -> (w541:sgl[])
                    n157 = Build Array(w540) -> (w537:sgl[][])
                  }
                  frame True {
                    n158 = call "8HP_Convert serial string to Eng vals.vi"("Serial buffer string (excluding FrameChar)"=w556) -> ("All vals"=w549:sgl[], "Pressures"=w547:sgl[][], "Gyration vector (deg / s)"=w550:sgl[], "External thermistor 0 temperature (deg C)"=w555:sgl, "External thermistor 1 temperature (deg C)"=w554:sgl, "Atmospheric pressure (mbar)"=w548:sgl, "Env. sensor die temperature (deg C)"=w553:sgl, "Relative humidity (%)"=w552:sgl, "Acceleration vector (g)"=w551:sgl[])  [unwired: 10 in]
                  }
                }
                "Pressures" <- w503
                "Acceleration vector (g)" <- w498
                "Gyration vector (deg / s)" <- w497
                "Atmospheric pressure (mbar)" <- w494
                "External thermistor 0 temperature (deg C)" <- w492
                "Env. sensor die temperature (deg C)" <- w500
                "Relative humidity (%)" <- w499
                "External thermistor 1 temperature (deg C)" <- w493
                n159 = case shown="True" w507 {
                  tunnel: w521 -> [w562 w579]
                  tunnel: [w562 w578] -> w520
                  tunnel: w519 -> [_ w577]
                  tunnel: w505 -> [_ w574]
                  tunnel: w518 -> [w560 w573]
                  tunnel: w517 -> [w561 w572]
                  tunnel: [w561 w571] -> w516
                  tunnel: [w560 w570] -> w515
                  tunnel: w513 -> [w559 w569]
                  tunnel: [w559 w568] -> w514
                  tunnel: w512 -> [w558 w567]
                  tunnel: w511 -> [_ w566]
                  tunnel: [w558 w565] -> w510
                  tunnel: w509 -> [w557 w564]
                  tunnel: [w557 w563] -> w508
                  frame False {
                  }
                  frame True {
                    n160 = Increment(x=w579) -> (x+1=w578:u32)
                    n161 = Quotient & Remainder(x=w578, y=w577) -> (x-y*floor(x/y)=w576:u32)  [unwired: 1 out]
                    n162 = Equal To 0?(x=w576) -> (x = 0?=w575:bool)
                    n163 = case shown="True" w575 {
                      tunnel: w574 -> [w587 _]
                      tunnel: w573 -> [w588 w601]
                      tunnel: w572 -> [w589 w600]
                      tunnel: [w589 w599] -> w571
                      tunnel: [w588 w598] -> w570
                      tunnel: w569 -> [w581 w593]
                      tunnel: [w580 sgl[][] []] -> w568
                      tunnel: w567 -> [w582 w596]
                      tunnel: w566 -> [w586 _]
                      tunnel: [w585 w596] -> w565
                      tunnel: w564 -> [w584 w595]
                      tunnel: [w583 sgl[] []] -> w563
                      frame False {
                        n164 = Add(x=w582, y=w586) -> (x+y=w585:sgl)
                        n165 = Build Array (concatenate)(w581, w587) -> (w580:sgl[][])
                        n166 = Build Array (concatenate)(w584, w582) -> (w583:sgl[])
                      }
                      frame True {
                        # "Write to disk every f samples (i.e. 1 s intervals)"
                        n167 = Transpose 2D Array(2D array=w593) -> (transposed array=w592:sgl[][])
                        n168 = Build Array (concatenate)(w595, w592) -> (w591:sgl[][])
                        n169 = Transpose 2D Array(2D array=w591) -> (transposed array=w590:sgl[][])
                        n170 = Array To Spreadsheet String(delimiter (Tab)="\t", array=w590, 3:"%.6f" ("format string")) -> (spreadsheet string=w604:string)
                        n171 = Write to Text File(file (use dialog)=w601, text=w604, error in=w600) -> (refnum out=w598:refnum<file>, error out=w599:errorcluster)  [unwired: 1 in, 1 out]
                      }
                    }
                  }
                }
                n172 = local write "Checksum ok"(w502) -> ()
                n173 = Index Array(array=w503, index (row)=0) -> (element=w506:sgl[])  [unwired: 1 in]
              }
            }
            n174 = Greater Or Equal?(x=w442, y=w444) -> (x >= y?=w443:bool)
            n175 = call <vilib>:"Clear Errors.vi"("error in (no error)"=w457, "specific error code to clear (0: all)"=1073676294) -> ("error out"=w456:errorcluster)  [unwired: 4 in, 1 out]
            n176 = local write "Error"(w456) -> ()
            n177 = Compound Arithmetic op=OR(w456, "Stop Data", w443) -> (w475:bool)
          }
          n178 = case shown="True" w405 {
            tunnel: [w428 w441] -> w415
            tunnel: w410 -> [w428 w433]
            tunnel: w409 -> [_ w434]
            tunnel: w392 -> [_ w432]
            tunnel: w391 -> [_ w431]
            frame False {
            }
            frame True {
              # "Write any remaining data to disk, then close file"
              n179 = Transpose 2D Array(2D array=w432) -> (transposed array=w438:sgl[][])
              n180 = Build Array (concatenate)(w431, w438) -> (w439:sgl[][])
              n181 = Transpose 2D Array(2D array=w439) -> (transposed array=w440:sgl[][])
              n182 = Array To Spreadsheet String(delimiter (Tab)="\t", array=w440, 3:"%.6f" ("format string")) -> (spreadsheet string=w435:string)
              n183 = Write to Text File(file (use dialog)=w434, text=w435, error in=w433) -> (refnum out=w430:refnum<file>, error out=w429:errorcluster)  [unwired: 1 in, 1 out]
              n184 = Close File(refnum=w430, error in=w429) -> (error out=w441:errorcluster)  [unwired: 1 out]
            }
          }
          n185 = Transpose 2D Array(2D array=w384) -> (transposed array=w386:sgl[][])
          n186 = Transpose 2D Array(2D array=w378) -> (transposed array=w387:sgl[][])
          n187 = Transpose 2D Array(2D array=w379) -> (transposed array=w388:sgl[][])
          n188 = Multiply(x=w395, y=sgl 2000.0) -> (x*y=w396:sgl)
          n189 = To Unsigned Long Integer(number=w396) -> (unsigned 32bit integer=w393:u32)
          n190 = Build Array (concatenate)(w386, w383, w382, w381, w380, w377, w387, w388) -> (w385:sgl[][])
          n191 = call "8HP_Send Cmd.vi"("Operation"=T2 "d" ("Combo Box"), "Port"=w402) -> ("Error Out"=w399:errorcluster, "Port out"=w400:refnum<visa-resource-name>)  [unwired: 2 in]
          n192 = call "Clear buffer.vi"("Error in"=w399, "dt for timeout (ms)"=w393, "VISA resource name in"=w400) -> ("Error out"=w397:errorcluster, "VISA resource name out"=w398:refnum<visa-resource-name>)  [unwired: 3 in]
          n193 = call "Close serial port.vi"("Error in"=w397, "VISA resource name"=w398) -> ("Error out"=w416:errorcluster)  [unwired: 9 in]
        }
      }
      n194 = local write "Stream enabled"(w306) -> ()
      n195 = Merge Errors(w302, w303, w301) -> (w300:errorcluster)
    }
    frame "d" {
      # "Disable USB streaming"
      n196 = flat-sequence {
        tunnel: [w619] -> w612
        tunnel: w611 -> [w619]
        tunnel: w605 -> [w618]
        tunnel: [w613] -> w606
        tunnel: w612 -> [w628]
        tunnel: [w627] -> w610
        tunnel: [TRUE] -> w607
        tunnel: w606 -> [w621]
        frame #0 {
          n197 = Reciprocal(x=w618) -> (1/x=w617:dbl)
          n198 = disable-structure shown="Disabled" {
            frame Disabled {
              n199 = local write "Main"(T1."Data stream" ("Main")) -> ()
            }
            frame Enabled {
            }
          }
          n200 = To Single Precision Float(number=w617) -> (single precision float=w614:sgl)
          n201 = Multiply(x=w614, y=sgl 2000.0) -> (x*y=w615:sgl)
          n202 = To Unsigned Long Integer(number=w615) -> (unsigned 32bit integer=w613:u32)
        }
        frame #1 {
          n203 = local read "COM port"() -> (w629:refnum<visa-resource-name>)
          n204 = call "Open serial port.vi"("timeout (ms)"=u32 5000, "VISA resource name"=w629) -> ("Error out"=w630:errorcluster, "VISA resource name out"=w631:refnum<visa-resource-name>)  [unwired: 8 in]
          n205 = call "8HP_Send Cmd.vi"("Error In"=w630, "Operation"=w628, "Port"=w631) -> ("Error Out"=w625:errorcluster, "Port out"=w623:refnum<visa-resource-name>)  [unwired: 1 in]
          n206 = call "Clear buffer.vi"("Error in"=w625, "dt for timeout (ms)"=w621, "VISA resource name in"=w623) -> ("Error out"=w624:errorcluster, "VISA resource name out"=w622:refnum<visa-resource-name>)  [unwired: 3 in]
          n207 = call "Close serial port.vi"("Error in"=w624, "VISA resource name"=w622) -> ("Error out"=w627:errorcluster)  [unwired: 9 in]
        }
      }
    }
    frame "F" {
      # "Set data rate"
      n208 = flat-sequence {
        tunnel: w641 -> [w644]
        tunnel: [w644] -> w640
        tunnel: w640 -> [w651]
        tunnel: [w650] -> w639
        tunnel: [w649] -> w638
        tunnel: [w714] -> w637
        tunnel: w639 -> [w714]
        tunnel: w638 -> [w712]
        tunnel: [w712] -> w634
        tunnel: [TRUE] -> w633
        frame #0 {
          n209 = local write "Returned data rate (Hz)"(u16 0 ("Returned data rate (Hz)")) -> ()
          n210 = local write "received"(FALSE ("sent")) -> ()
          n211 = local write "Main"(T1."Data rate" ("Main")) -> ()
          n212 = local write "sent"(FALSE ("sent")) -> ()
        }
        frame #1 {
          # "to LE"
          n213 = local read "Set data rate (Hz)"() -> (w647:u8)
          n214 = case shown="14, Default" w647 {
            tunnel: [1.0 2.0 4.0 5.0 8.0 10.0 16.0 20.0 25.0 32.0 40.0 50.0 64.0 80.0 100.0 125.0 160.0 200.0 250.0 320.0 400.0 500.0 625.0 800.0 1000.0] -> w650
            tunnel: [u8 0 u8 0 u8 0 u8 0 u8 0 u8 0 u8 0 u8 0 u8 1 u8 1 u8 1 u8 2 u8 2 u8 2 u8 3 u8 3 u8 3 u8 4 u8 4 u8 4 u8 5 u8 5 u8 6 u8 6 u8 6] -> _
            frame 0 {
            }
            frame 1 {
            }
            frame 2 {
            }
            frame 3 {
            }
            frame 4 {
            }
            frame 5 {
            }
            frame 6 {
            }
            frame 7 {
            }
            frame 8 {
            }
            frame 9 {
            }
            frame 10 {
            }
            frame 11 {
            }
            frame 12 {
            }
            frame 13 {
            }
            frame 14, Default {
            }
            frame 15 {
            }
            frame 16 {
            }
            frame 17 {
            }
            frame 18 {
            }
            frame 19 {
            }
            frame 20 {
            }
            frame 21 {
            }
            frame 22 {
            }
            frame 23 {
            }
            frame 24 {
            }
          }
          n215 = local read "COM port"() -> (w654:refnum<visa-resource-name>)
          n216 = To Unsigned Word Integer(number=w650) -> (unsigned 16bit integer=w658:u16)
          n217 = Type Cast(type="", x=w658) -> (*(type *) &x=w660:string)
          n218 = call "Open serial port.vi"("timeout (ms)"=u32 5000, "VISA resource name"=w654) -> ("Error out"=w655:errorcluster, "VISA resource name out"=w656:refnum<visa-resource-name>)  [unwired: 8 in]
          n219 = Reverse String(1:w660) -> (0:w648:string)
          n220 = call "8HP_Send Cmd + Data.vi"("Error In"=w655, "Data"=w648, "Operation"=w651, "Port"=w656) -> ("Error Out"=w652:errorcluster, "Port out"=w653:refnum<visa-resource-name>)  [unwired: 1 in]
          n221 = call "Close serial port.vi"("Error in"=w652, "VISA resource name"=w653) -> ("Error out"=w649:errorcluster)  [unwired: 9 in]
        }
        frame #2 {
          n222 = Unbundle By Name(w712) -> ("status"=w713:bool)
          n223 = Not(x=w713) -> (.not. x?=→"sent":bool)
        }
      }
    }
    frame "f" {
      # "Get data rate"
      n224 = flat-sequence {
        tunnel: w724 -> [w727]
        tunnel: [w727] -> w723
        tunnel: w723 -> [w737]
        tunnel: [w740] -> w722
        tunnel: [w742] -> w721
        tunnel: [w749] -> w720
        tunnel: w722 -> [w749]
        tunnel: w721 -> [w747]
        tunnel: [w747] -> w717
        tunnel: [TRUE] -> w716
        frame #0 {
          n225 = local write "received"(FALSE ("sent")) -> ()
          n226 = local write "Main"(T1."Data rate" ("Main")) -> ()
          n227 = local write "sent"(FALSE ("sent")) -> ()
        }
        frame #1 {
          # "to BE"
          n228 = local read "COM port"() -> (w743:refnum<visa-resource-name>)
          n229 = call "Open serial port.vi"("timeout (ms)"=u32 5000, "VISA resource name"=w743) -> ("Error out"=w738:errorcluster, "VISA resource name out"=w739:refnum<visa-resource-name>)  [unwired: 8 in]
          n230 = call "8HP_Send Cmd.vi"("Error In"=w738, "Operation"=w737, "Port"=w739) -> ("Error Out"=w735:errorcluster, "Port out"=w734:refnum<visa-resource-name>)  [unwired: 1 in]
          n231 = VISA Read(VISA resource name=w734, byte count=u32 2, error in (no error)=w735) -> (VISA resource name out=w732:refnum<visa-resource-name>, read buffer=w731:string, error out=w733:errorcluster)  [unwired: 1 out]
          n232 = Reverse String(1:w731) -> (0:w741:string)
          n233 = call "Close serial port.vi"("Error in"=w733, "VISA resource name"=w732) -> ("Error out"=w742:errorcluster)  [unwired: 9 in]
          n234 = Type Cast(type=u16 0 ("byte count"), x=w741) -> (*(type *) &x=w729:u16)
          "Returned data rate (Hz)" <- w729
          n235 = To Double Precision Float(number=w729) -> (double precision float=w740:dbl)
        }
        frame #2 {
          n236 = Unbundle By Name(w747) -> ("status"=w748:bool)
          n237 = Not(x=w748) -> (.not. x?=→"received":bool)
        }
      }
    }
    frame "N" {
      # "Get serial number"
      n238 = flat-sequence {
        tunnel: w753 -> [w759]
        tunnel: [w759] -> w752
        tunnel: [TRUE] -> w756
        tunnel: w752 -> [w765]
        tunnel: [w764] -> w751
        frame #0 {
          n239 = local write "Main"(T1."Action" ("Main")) -> ()
          "Serial number" <- sgl 0.0 ("Numeric")
        }
        frame #1 {
          # "to BE"
          n240 = local read "COM port"() -> (w766:refnum<visa-resource-name>)
          n241 = call "Open serial port.vi"("timeout (ms)"=u32 5000, "VISA resource name"=w766) -> ("Error out"=w773:errorcluster, "VISA resource name out"=w774:refnum<visa-resource-name>)  [unwired: 8 in]
          n242 = call "8HP_Send Cmd.vi"("Error In"=w773, "Operation"=w765, "Port"=w774) -> ("Error Out"=w771:errorcluster, "Port out"=w772:refnum<visa-resource-name>)  [unwired: 1 in]
          n243 = VISA Read(VISA resource name=w772, byte count=u32 4, error in (no error)=w771) -> (VISA resource name out=w769:refnum<visa-resource-name>, read buffer=w761:string, error out=w768:errorcluster)  [unwired: 1 out]
          n244 = call "Close serial port.vi"("Error in"=w768, "VISA resource name"=w769) -> ("Error out"=w764:errorcluster)  [unwired: 9 in]
          n245 = Reverse String(1:w761) -> (0:w762:string)
          n246 = Type Cast(type=sgl 0.0 ("byte count"), x=w762) -> (*(type *) &x=w760:sgl)
          n247 = local write "Serial number"(w760) -> ()
        }
      }
    }
    frame "X" {
      # "Exit"
    }
    frame Default {
    }
  }
  "All samples out" <- w2
  n248 = Merge Errors(w11, w10, w9) -> (w8:errorcluster)
  n249 = call <vilib>:"Clear Errors.vi"("error in (no error)"=w8, "specific error code to clear (0: all)"=1073676294) -> ("error out"=w5:errorcluster)  [unwired: 4 in, 1 out]
  n250 = local write "Error"(w5) -> ()
  n251 = Release Queue(queue=w6, error in (no error)=w5) -> (error out=→"Error":errorcluster)  [unwired: 1 in, 2 out]
